vi "Read Database.lvclass.vi"(8 "error in (no error)":errorcluster, 11 "Field in":refnum<class "Field.lvclass">) -> (0 "error out":errorcluster, 2 "Database.lvclass":refnum<class "Database.lvclass">, 3 "Field out":refnum<class "Field.lvclass">)   [LabVIEW 2020, in "Field.lvclass"]
uses:
  Field.lvclass
  Database.lvclass
  Field.lvclass/Field.ctl
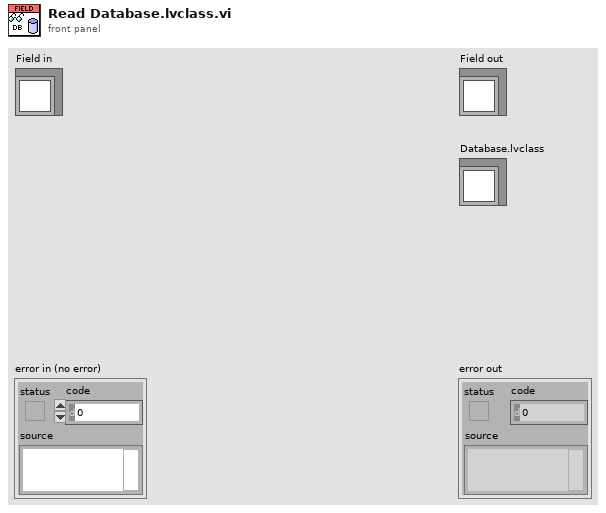
[diagram p1: front panel]
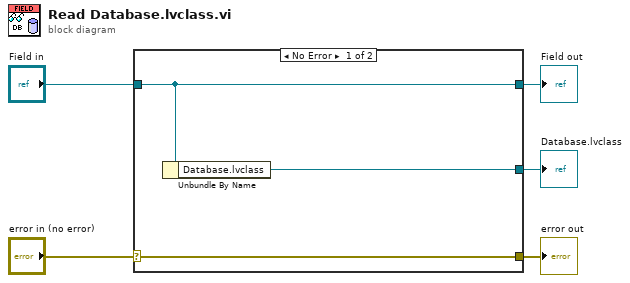
[diagram p0: block diagram]
diagram:
  n1 = case shown="No Error" "error in (no error)" {
    selector: "error in (no error)" -> [w8 w9]
    tunnel: [w8 w9] -> w4
    tunnel: [w7 w10] -> w2
    tunnel: "Field in" -> [w7 w10]
    tunnel: [w6 _] -> w1
    frame No Error {
      n2 = Unbundle By Name(w7) -> ("Database.lvclass"=w6:refnum<class "Database.lvclass">)
    }
    frame Error {
    }
  }
  "error out" <- w4
  "Field out" <- w2
  "Database.lvclass" <- w1
